vi "Set SelectionMode.vi"(8 "error in":errorcluster, 10 "SelectionMode":i32(ring)=2 items=["Cell"=1, "Row"=2, "Column"=3], 11 "Sourcegrid in":refnum<class "SourceGrid.lvclass">) -> (0 "error out":errorcluster, 3 "Sourcegrid out":refnum<class "SourceGrid.lvclass">)   [LabVIEW 2024, in "SourceGrid.lvlib" / "SourceGrid.lvclass"]
uses:
  SourceGrid.lvclass
  SourceGrid.lvclass/SourceGrid.ctl
  D:/git/Sourcegrid-LabVIEW/dll/SourceGrid.dll
  dll/SourceGrid.dll
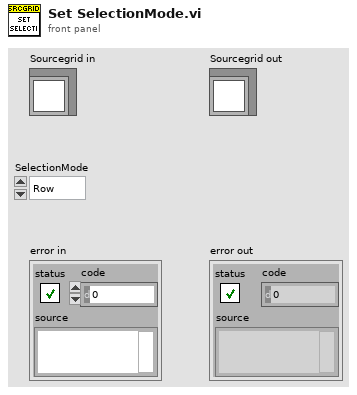
[diagram p1: front panel]
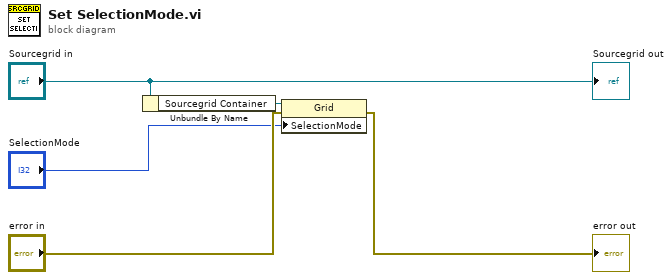
[diagram p0: block diagram]
diagram:
  n1 = Unbundle By Name("Sourcegrid in") -> ("Sourcegrid Container"=w2:refnum<k24>)
  n2 = property class="Grid"(reference=w2, error in="error in", "SelectionMode"="SelectionMode") -> (error out=→"error out":errorcluster)  [unwired: 1 out]
  "Sourcegrid out" <- "Sourcegrid in"
